vi "StartCCLM.vi"(0 "VISA resource name":refnum<visa-resource-name>, 5 "Device Control-In 2":T1={"Stimulation Parameters"={"Amplitude (mA)"={"A1"=1, "A2"=0, "A3"=0, "A4"=0, "A5"=0, "A6"=0, "A7"=0, "A8"=0}, "Pulse Width (µs)"={"PW1"=20, "PW2"=20, "PW3"=20, "PW4"=20, "PW5"=20, "PW6"=20, "PW7"=20, "PW8"=20}, "Stimulation Mode"={"M1"=0, "M2"=0, "M3"=0, "M4"=0, "M5"=0, "M6"=0, "M7"=0, "M8"=0}}, "Waveform Parameters"={"Low Frequency Factor"=0, "Main Stim Interval [ms]"=8.0, "Interpulse Interval [ms]"=0, "Channel Execution"=0}, "Active channels"={"C1"=FALSE, "C2"=FALSE, "C3"=FALSE, "C4"=FALSE, "C5"=FALSE, "C6"=FALSE, "C7"=FALSE, "C8"=FALSE}, "LF Active Channels"={"LF1"=FALSE, "LF2"=FALSE, "LF3"=FALSE, "LF4"=FALSE, "LF5"=FALSE, "LF6"=FALSE, "LF7"=FALSE, "LF8"=FALSE}, "Device Control"={"VISA resource name"=""}} {"Stimulation Parameters"."Amplitude (mA)"."A1" max=130; "Stimulation Parameters"."Amplitude (mA)"."A2" max=130; "Stimulation Parameters"."Amplitude (mA)"."A3" max=130; "Stimulation Parameters"."Amplitude (mA)"."A4" max=130; "Stimulation Parameters"."Amplitude (mA)"."A5" max=130; "Stimulation Parameters"."Amplitude (mA)"."A6" max=130; "Stimulation Parameters"."Amplitude (mA)"."A7" max=130; "Stimulation Parameters"."Amplitude (mA)"."A8" max=130; "Stimulation Parameters"."Pulse Width (µs)"."PW1" min=20 max=500; "Stimulation Parameters"."Pulse Width (µs)"."PW2" min=20 max=500; "Stimulation Parameters"."Pulse Width (µs)"."PW3" min=20 max=500; "Stimulation Parameters"."Pulse Width (µs)"."PW4" min=20 max=500; "Stimulation Parameters"."Pulse Width (µs)"."PW5" min=20 max=500; "Stimulation Parameters"."Pulse Width (µs)"."PW6" min=20 max=500; "Stimulation Parameters"."Pulse Width (µs)"."PW7" min=20 max=500; "Stimulation Parameters"."Pulse Width (µs)"."PW8" min=20 max=500; "Stimulation Parameters"."Stimulation Mode"."M8" items=["Singlet", "Doublet", "Triplet"]; "Stimulation Parameters"."Stimulation Mode"."M7" items=["Singlet", "Doublet", "Triplet"]; "Stimulation Parameters"."Stimulation Mode"."M6" items=["Singlet", "Doublet", "Triplet"]; "Stimulation Parameters"."Stimulation Mode"."M5" items=["Singlet", "Doublet", "Triplet"]; "Stimulation Parameters"."Stimulation Mode"."M4" items=["Singlet", "Doublet", "Triplet"]; "Stimulation Parameters"."Stimulation Mode"."M3" items=["Singlet", "Doublet", "Triplet"]; "Stimulation Parameters"."Stimulation Mode"."M2" items=["Singlet", "Doublet", "Triplet"]; "Stimulation Parameters"."Stimulation Mode"."M1" items=["Singlet", "Doublet", "Triplet"]; "Waveform Parameters"."Channel Execution" items=["Fixed Interval", "ASAP"]}, 7 "StimInitializationEnable":bool=TRUE, 11 "error in (no error)":errorcluster) -> (4 "VISA resource name out":refnum<visa-resource-name>, 8 "Stimulation Started":bool=TRUE, 15 "error out":errorcluster)   [LabVIEW 2020]
uses:
  Type Defs/rs2_ctrl_panel.ctl
panel:
  in  "Boolean":bool
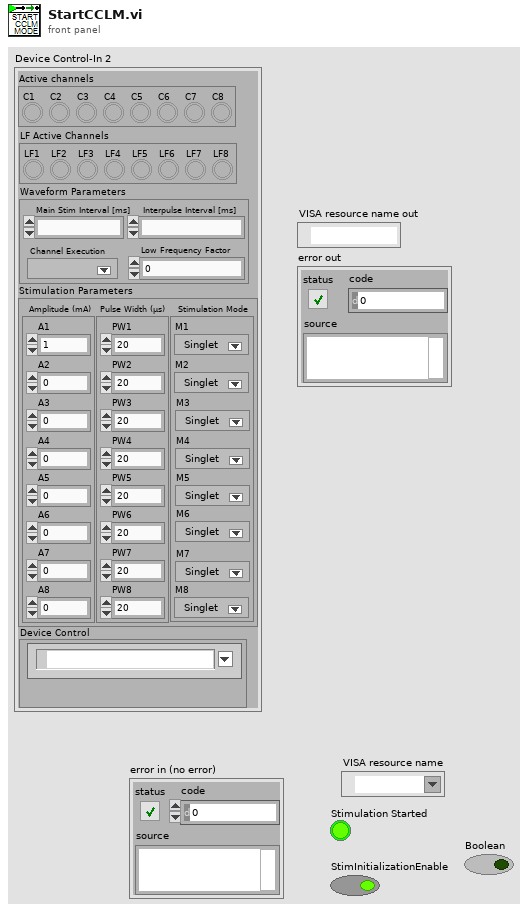
[diagram p1: front panel]
types:
  T1 = typedef "rs2_ctrl_panel.ctl" = cluster{"Stimulation Parameters":cluster{"Amplitude (mA)":cluster{"A1":u8, "A2":u8, "A3":u8, "A4":u8, "A5":u8, "A6":u8, "A7":u8, "A8":u8}, "Pulse Width (µs)":cluster{"PW1":u16, "PW2":u16, "PW3":u16, "PW4":u16, "PW5":u16, "PW6":u16, "PW7":u16, "PW8":u16}, "Stimulation Mode":cluster{"M1":u8, "M2":u8, "M3":u8, "M4":u8, "M5":u8, "M6":u8, "M7":u8, "M8":u8}}, "Waveform Parameters":cluster{"Low Frequency Factor":u8, "Main Stim Interval [ms]":fxp<+,32,11>, "Interpulse Interval [ms]":u8, "Channel Execution":u8}, "Active channels":cluster{"C1":bool, "C2":bool, "C3":bool, "C4":bool, "C5":bool, "C6":bool, "C7":bool, "C8":bool}, "LF Active Channels":cluster{"LF1":bool, "LF2":bool, "LF3":bool, "LF4":bool, "LF5":bool, "LF6":bool, "LF7":bool, "LF8":bool}, "Device Control":cluster{"VISA resource name":refnum<visa-resource-name>}}
  T2 = cluster{"C1":bool, "C2":bool, "C3":bool, "C4":bool, "C5":bool, "C6":bool, "C7":bool, "C8":bool}
  T3 = cluster{"Amplitude (mA)":cluster{"A1":u8, "A2":u8, "A3":u8, "A4":u8, "A5":u8, "A6":u8, "A7":u8, "A8":u8}, "Pulse Width (µs)":cluster{"PW1":u16, "PW2":u16, "PW3":u16, "PW4":u16, "PW5":u16, "PW6":u16, "PW7":u16, "PW8":u16}, "Stimulation Mode":cluster{"M1":u8, "M2":u8, "M3":u8, "M4":u8, "M5":u8, "M6":u8, "M7":u8, "M8":u8}}
  T4 = cluster{"A1":u8, "A2":u8, "A3":u8, "A4":u8, "A5":u8, "A6":u8, "A7":u8, "A8":u8}
  T5 = cluster{"PW1":u16, "PW2":u16, "PW3":u16, "PW4":u16, "PW5":u16, "PW6":u16, "PW7":u16, "PW8":u16}
  T6 = cluster{"M1":u8, "M2":u8, "M3":u8, "M4":u8, "M5":u8, "M6":u8, "M7":u8, "M8":u8}
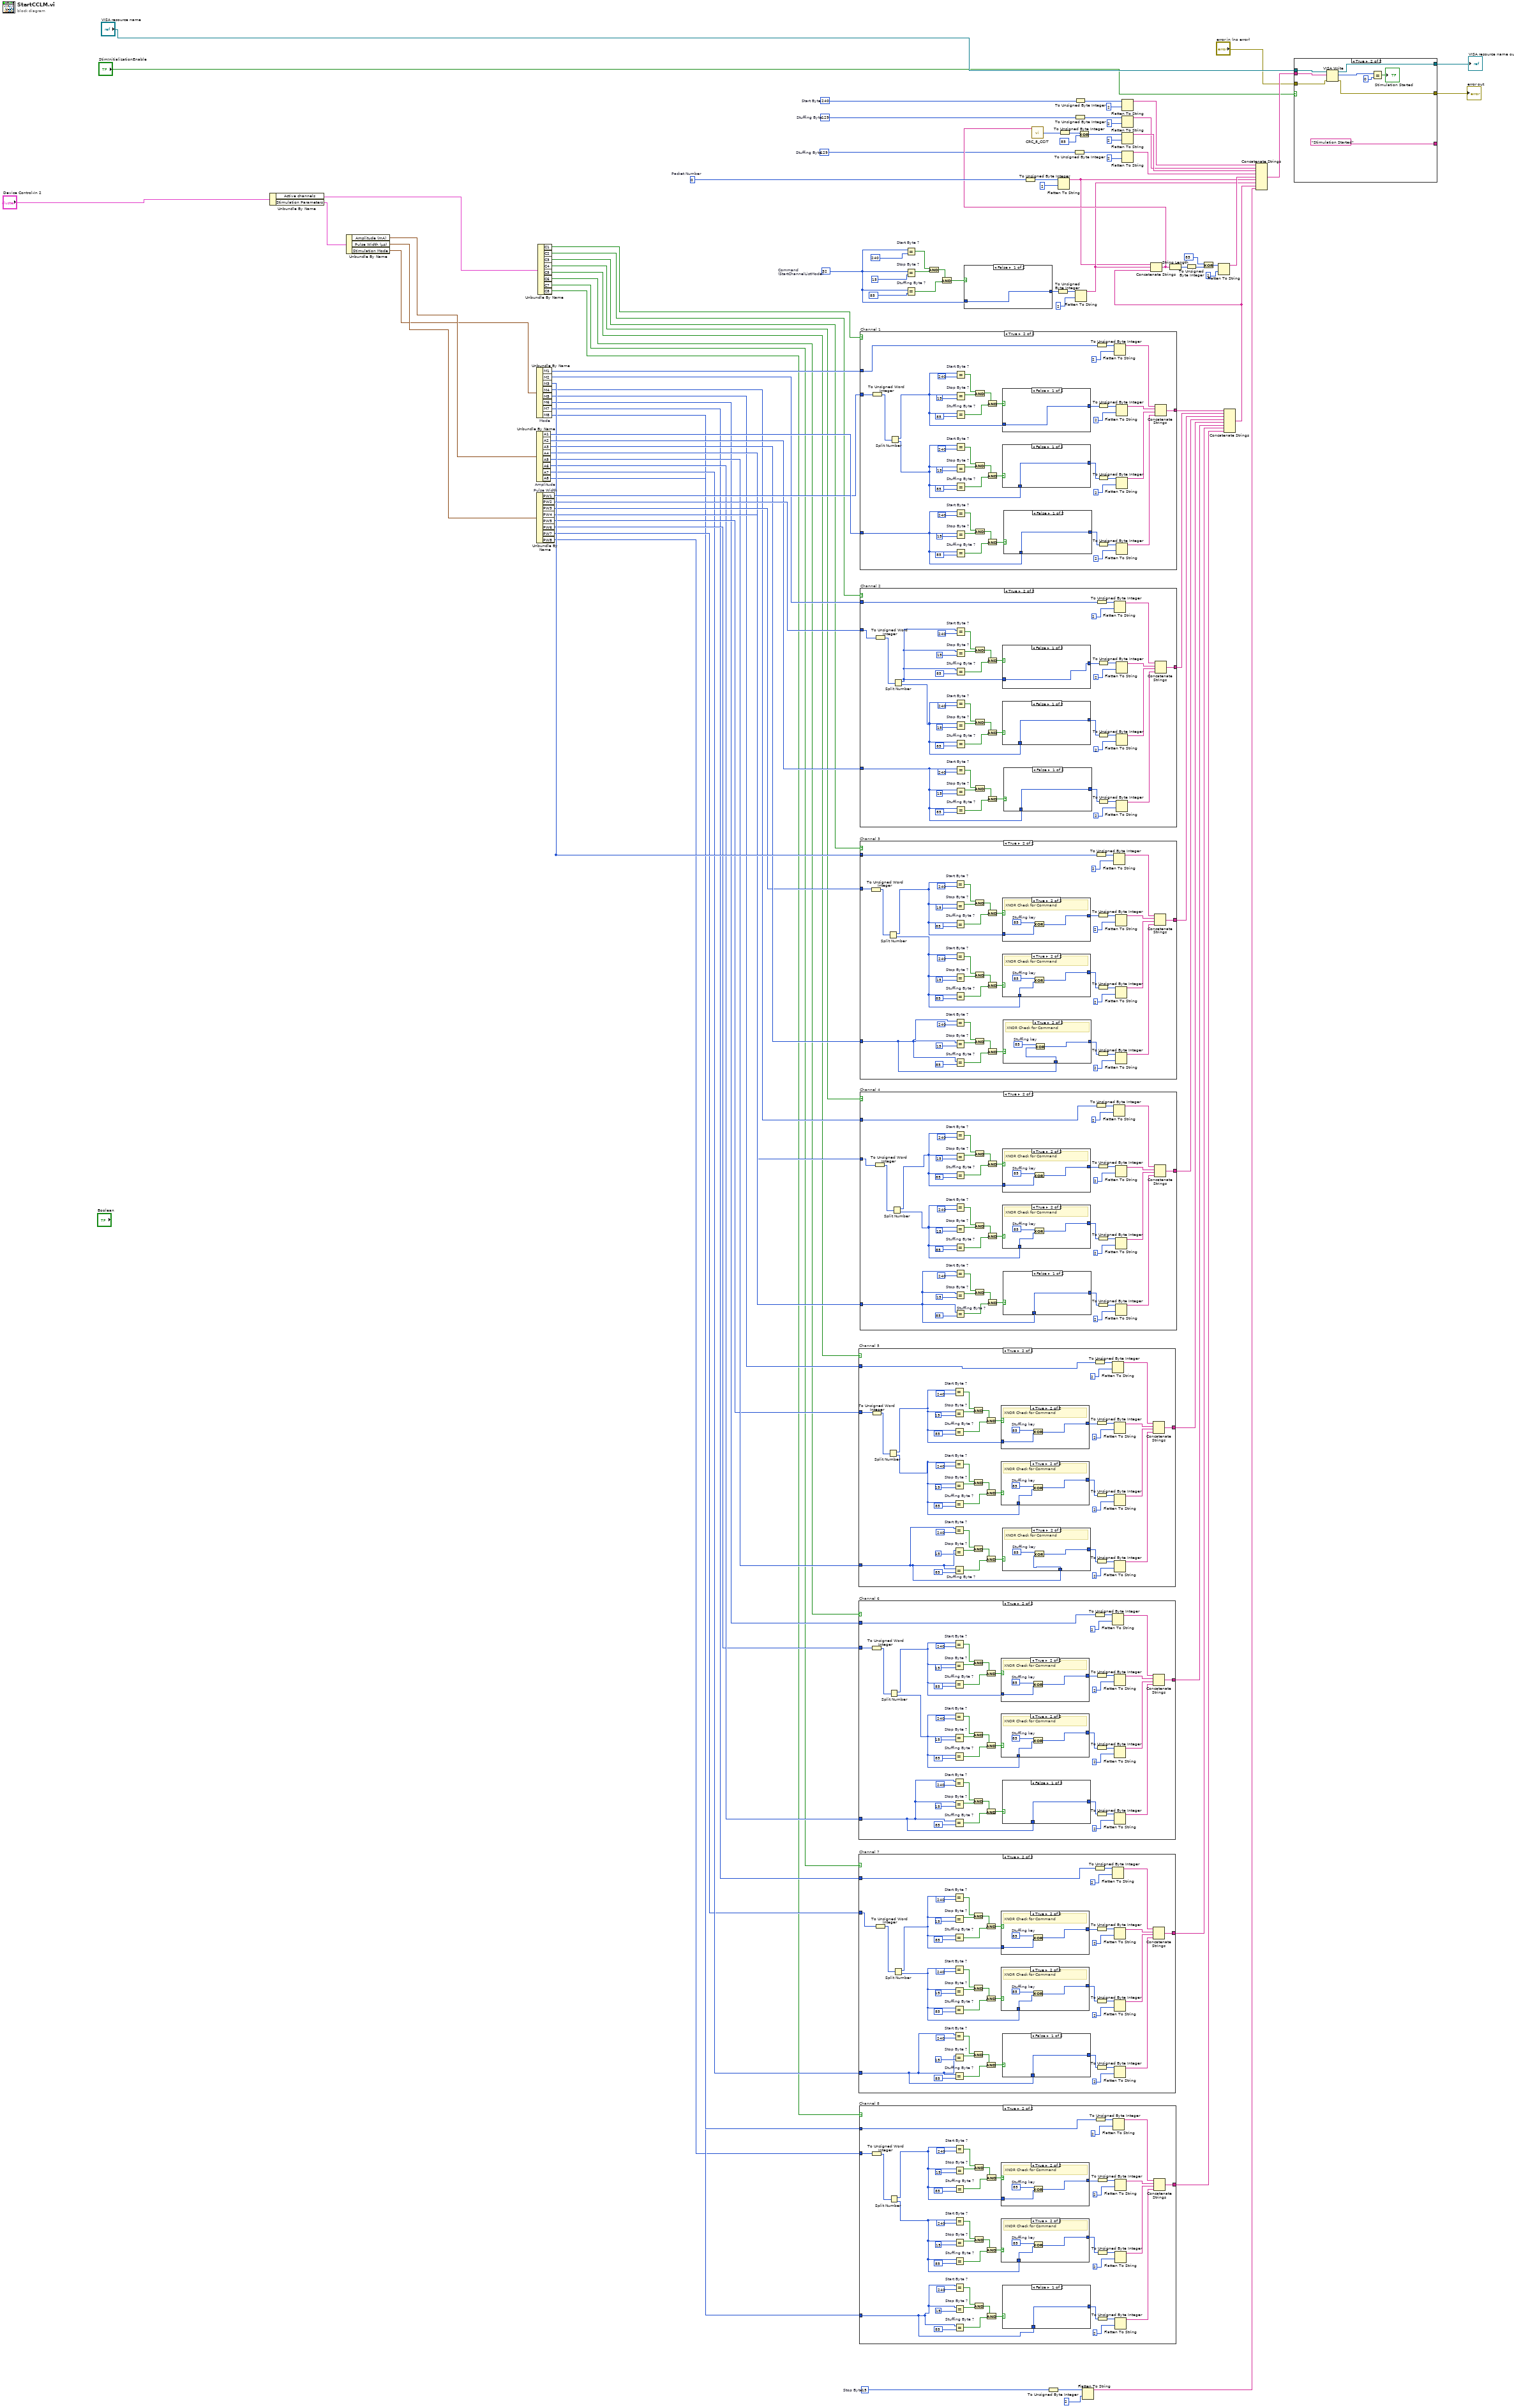
[diagram p0: block diagram]
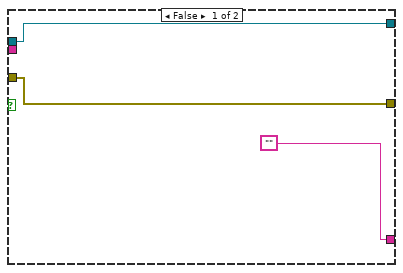
[diagram p2: hidden frame]
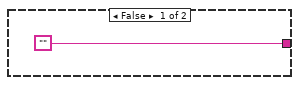
[diagram p3: hidden frame]
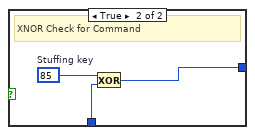
[diagram p4: hidden frame]
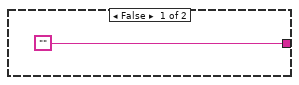
[diagram p7: hidden frame]
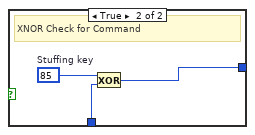
[diagram p8: hidden frame]
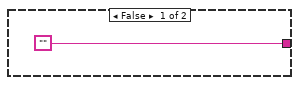
[diagram p11: hidden frame]
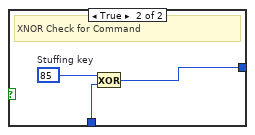
[diagram p12: hidden frame]
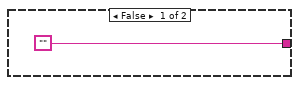
[diagram p15: hidden frame]
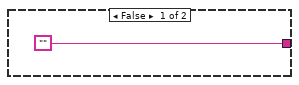
[diagram p19: hidden frame]
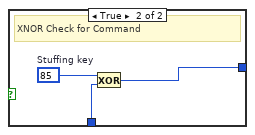
[diagram p20: hidden frame]
diagram:
  w99 = u8 0  # Packet Number
  w63 = 15  # Stop Byte
  w66 = 129  # Stuffing Byte
  w67 = 129  # Stuffing Byte
  w65 = 240  # Start Byte
  w81 = 32  # Command (StartChannelListMode)
  n1 = Unbundle By Name("Device Control-In 2") -> ("Active channels"=w5:T2, "Stimulation Parameters"=w4:T3)
  n2 = Unbundle By Name(w4) -> ("Amplitude (mA)"=w3:T4, "Pulse Width (µs)"=w2:T5, "Stimulation Mode"=w1:T6)
  n3 = Unbundle By Name "Mode"(w1) -> ("M1"=w41:u8, "M2"=w40:u8, "M3"=w37:u8, "M4"=w34:u8, "M5"=w31:u8, "M6"=w28:u8, "M7"=w25:u8, "M8"=w22:u8)
  n4 = Unbundle By Name "Amplitude"(w3) -> ("A1"=w43:u8, "A2"=w38:u8, "A3"=w36:u8, "A4"=w33:u8, "A5"=w30:u8, "A6"=w27:u8, "A7"=w24:u8, "A8"=w21:u8)
  n5 = Unbundle By Name "Pulse Width"(w2) -> ("PW1"=w42:u16, "PW2"=w39:u16, "PW3"=w35:u16, "PW4"=w32:u16, "PW5"=w29:u16, "PW6"=w26:u16, "PW7"=w23:u16, "PW8"=w20:u16)
  n6 = Unbundle By Name(w5) -> ("C1"=w19:bool, "C2"=w18:bool, "C3"=w17:bool, "C4"=w16:bool, "C5"=w15:bool, "C6"=w14:bool, "C7"=w13:bool, "C8"=w12:bool)
  n7 = case "Channel 5" shown="True" w15 {
    tunnel: ["" w107] -> w47
    tunnel: w31 -> [_ w106]
    tunnel: w30 -> [_ w101]
    tunnel: w29 -> [_ w104]
    frame False {
    }
    frame True {
      n8 = To Unsigned Word Integer(number=w104) -> (unsigned 16bit integer=w105:u16)
      n9 = Split Number(x=w105) -> (hi(x)=w103:u8, lo(x)=w102:u8)
      n10 = Equal? "Start Byte ?"(x=w103, y=240 ("IntAck")) -> (x = y?=w136:bool)
      n11 = Equal? "Stop Byte ?"(x=w103, y=15 ("IntAck")) -> (x = y?=w137:bool)
      n12 = Equal? "Stuffing Byte ?"(x=w103, y=85 ("IntAck")) -> (x = y?=w139:bool)
      n13 = Equal? "Start Byte ?"(x=w102, y=240 ("IntAck")) -> (x = y?=w125:bool)
      n14 = Equal? "Stop Byte ?"(x=w102, y=15 ("IntAck")) -> (x = y?=w126:bool)
      n15 = Equal? "Stuffing Byte ?"(x=w102, y=85 ("IntAck")) -> (x = y?=w128:bool)
      n16 = Equal? "Start Byte ?"(x=w101, y=240 ("IntAck")) -> (x = y?=w114:bool)
      n17 = Equal? "Stop Byte ?"(x=w101, y=15 ("IntAck")) -> (x = y?=w115:bool)
      n18 = Equal? "Stuffing Byte ?"(x=w101, y=85 ("IntAck")) -> (x = y?=w117:bool)
      n19 = And(x=w136, y=w137) -> (x .and. y?=w138:bool)
      n20 = And(x=w125, y=w126) -> (x .and. y?=w127:bool)
      n21 = And(x=w114, y=w115) -> (x .and. y?=w116:bool)
      n22 = And(x=w138, y=w139) -> (x .and. y?=w140:bool)
      n23 = And(x=w127, y=w128) -> (x .and. y?=w129:bool)
      n24 = And(x=w116, y=w117) -> (x .and. y?=w118:bool)
      n25 = case shown="True" w140 {
        tunnel: w103 -> [w155 w156]
        tunnel: [w155 w157] -> w145
        frame False {
        }
        frame True {
          w158 = 85  # Stuffing key
          # "XNOR Check for Command"
          n26 = Exclusive Or(1:w156, 2:w158) -> (0:w157:i32)
        }
      }
      n27 = case shown="True" w129 {
        tunnel: w102 -> [w151 w152]
        tunnel: [w151 w153] -> w134
        frame False {
        }
        frame True {
          w154 = 85  # Stuffing key
          # "XNOR Check for Command"
          n28 = Exclusive Or(1:w152, 2:w154) -> (0:w153:i32)
        }
      }
      n29 = case shown="True" w118 {
        tunnel: [w147 w149] -> w123
        tunnel: w101 -> [w147 w148]
        frame False {
        }
        frame True {
          w150 = 85  # Stuffing key
          # "XNOR Check for Command"
          n30 = Exclusive Or(1:w148, 2:w150) -> (0:w149:i32)
        }
      }
      n31 = To Unsigned Byte Integer(number=w106) -> (unsigned 8bit integer=w113:u8)
      n32 = To Unsigned Byte Integer(number=w145) -> (unsigned 8bit integer=w146:u8)
      n33 = To Unsigned Byte Integer(number=w134) -> (unsigned 8bit integer=w135:u8)
      n34 = To Unsigned Byte Integer(number=w123) -> (unsigned 8bit integer=w124:u8)
      n35 = Flatten To String(anything=w113, byte order (0:big-endian, network order)=2) -> (data string=w111:string)  [unwired: 2 in, 2 out]
      n36 = Flatten To String(anything=w146, byte order (0:big-endian, network order)=2) -> (data string=w110:string)  [unwired: 2 in, 2 out]
      n37 = Flatten To String(anything=w135, byte order (0:big-endian, network order)=2) -> (data string=w109:string)  [unwired: 2 in, 2 out]
      n38 = Flatten To String(anything=w124, byte order (0:big-endian, network order)=2) -> (data string=w108:string)  [unwired: 2 in, 2 out]
      n39 = Concatenate Strings(w111, w110, w109, w108) -> (w107:string)
    }
  }
  n40 = case "Channel 6" shown="True" w14 {
    tunnel: ["" w166] -> w46
    tunnel: w26 -> [_ w163]
    tunnel: w27 -> [_ w160]
    tunnel: w28 -> [_ w165]
    frame False {
    }
    frame True {
      n41 = To Unsigned Word Integer(number=w163) -> (unsigned 16bit integer=w164:u16)
      n42 = Split Number(x=w164) -> (hi(x)=w162:u8, lo(x)=w161:u8)
      n43 = Equal? "Start Byte ?"(x=w162, y=240 ("IntAck")) -> (x = y?=w195:bool)
      n44 = Equal? "Stop Byte ?"(x=w162, y=15 ("IntAck")) -> (x = y?=w196:bool)
      n45 = Equal? "Stuffing Byte ?"(x=w162, y=85 ("IntAck")) -> (x = y?=w198:bool)
      n46 = Equal? "Start Byte ?"(x=w161, y=240 ("IntAck")) -> (x = y?=w184:bool)
      n47 = Equal? "Stop Byte ?"(x=w161, y=15 ("IntAck")) -> (x = y?=w185:bool)
      n48 = Equal? "Stuffing Byte ?"(x=w161, y=85 ("IntAck")) -> (x = y?=w187:bool)
      n49 = Equal? "Start Byte ?"(x=w160, y=240 ("IntAck")) -> (x = y?=w173:bool)
      n50 = Equal? "Stop Byte ?"(x=w160, y=15 ("IntAck")) -> (x = y?=w174:bool)
      n51 = Equal? "Stuffing Byte ?"(x=w160, y=85 ("IntAck")) -> (x = y?=w176:bool)
      n52 = And(x=w195, y=w196) -> (x .and. y?=w197:bool)
      n53 = And(x=w184, y=w185) -> (x .and. y?=w186:bool)
      n54 = And(x=w173, y=w174) -> (x .and. y?=w175:bool)
      n55 = And(x=w197, y=w198) -> (x .and. y?=w199:bool)
      n56 = And(x=w186, y=w187) -> (x .and. y?=w188:bool)
      n57 = And(x=w175, y=w176) -> (x .and. y?=w177:bool)
      n58 = case shown="True" w199 {
        tunnel: w162 -> [w214 w215]
        tunnel: [w214 w216] -> w204
        frame False {
        }
        frame True {
          w217 = 85  # Stuffing key
          # "XNOR Check for Command"
          n59 = Exclusive Or(1:w215, 2:w217) -> (0:w216:i32)
        }
      }
      n60 = case shown="True" w188 {
        tunnel: w161 -> [w210 w211]
        tunnel: [w210 w212] -> w193
        frame False {
        }
        frame True {
          w213 = 85  # Stuffing key
          # "XNOR Check for Command"
          n61 = Exclusive Or(1:w211, 2:w213) -> (0:w212:i32)
        }
      }
      n62 = case shown="False" w177 {
        tunnel: [w206 w208] -> w182
        tunnel: w160 -> [w206 w207]
        frame False {
        }
        frame True {
          w209 = 85  # Stuffing key
          # "XNOR Check for Command"
          n63 = Exclusive Or(1:w207, 2:w209) -> (0:w208:i32)
        }
      }
      n64 = To Unsigned Byte Integer(number=w165) -> (unsigned 8bit integer=w172:u8)
      n65 = To Unsigned Byte Integer(number=w204) -> (unsigned 8bit integer=w205:u8)
      n66 = To Unsigned Byte Integer(number=w193) -> (unsigned 8bit integer=w194:u8)
      n67 = To Unsigned Byte Integer(number=w182) -> (unsigned 8bit integer=w183:u8)
      n68 = Flatten To String(anything=w172, byte order (0:big-endian, network order)=2) -> (data string=w170:string)  [unwired: 2 in, 2 out]
      n69 = Flatten To String(anything=w205, byte order (0:big-endian, network order)=2) -> (data string=w169:string)  [unwired: 2 in, 2 out]
      n70 = Flatten To String(anything=w194, byte order (0:big-endian, network order)=2) -> (data string=w168:string)  [unwired: 2 in, 2 out]
      n71 = Flatten To String(anything=w183, byte order (0:big-endian, network order)=2) -> (data string=w167:string)  [unwired: 2 in, 2 out]
      n72 = Concatenate Strings(w170, w169, w168, w167) -> (w166:string)
    }
  }
  n73 = case "Channel 7" shown="True" w13 {
    tunnel: ["" w225] -> w45
    tunnel: w23 -> [_ w222]
    tunnel: w24 -> [_ w219]
    tunnel: w25 -> [_ w224]
    frame False {
    }
    frame True {
      n74 = To Unsigned Word Integer(number=w222) -> (unsigned 16bit integer=w223:u16)
      n75 = Split Number(x=w223) -> (hi(x)=w221:u8, lo(x)=w220:u8)
      n76 = Equal? "Start Byte ?"(x=w221, y=240 ("IntAck")) -> (x = y?=w254:bool)
      n77 = Equal? "Stop Byte ?"(x=w221, y=15 ("IntAck")) -> (x = y?=w255:bool)
      n78 = Equal? "Stuffing Byte ?"(x=w221, y=85 ("IntAck")) -> (x = y?=w257:bool)
      n79 = Equal? "Start Byte ?"(x=w220, y=240 ("IntAck")) -> (x = y?=w243:bool)
      n80 = Equal? "Stop Byte ?"(x=w220, y=15 ("IntAck")) -> (x = y?=w244:bool)
      n81 = Equal? "Stuffing Byte ?"(x=w220, y=85 ("IntAck")) -> (x = y?=w246:bool)
      n82 = Equal? "Start Byte ?"(x=w219, y=240 ("IntAck")) -> (x = y?=w232:bool)
      n83 = Equal? "Stop Byte ?"(x=w219, y=15 ("IntAck")) -> (x = y?=w233:bool)
      n84 = Equal? "Stuffing Byte ?"(x=w219, y=85 ("IntAck")) -> (x = y?=w235:bool)
      n85 = And(x=w254, y=w255) -> (x .and. y?=w256:bool)
      n86 = And(x=w243, y=w244) -> (x .and. y?=w245:bool)
      n87 = And(x=w232, y=w233) -> (x .and. y?=w234:bool)
      n88 = And(x=w256, y=w257) -> (x .and. y?=w258:bool)
      n89 = And(x=w245, y=w246) -> (x .and. y?=w247:bool)
      n90 = And(x=w234, y=w235) -> (x .and. y?=w236:bool)
      n91 = case shown="True" w258 {
        tunnel: w221 -> [w273 w274]
        tunnel: [w273 w275] -> w263
        frame False {
        }
        frame True {
          w276 = 85  # Stuffing key
          # "XNOR Check for Command"
          n92 = Exclusive Or(1:w274, 2:w276) -> (0:w275:i32)
        }
      }
      n93 = case shown="True" w247 {
        tunnel: w220 -> [w269 w270]
        tunnel: [w269 w271] -> w252
        frame False {
        }
        frame True {
          w272 = 85  # Stuffing key
          # "XNOR Check for Command"
          n94 = Exclusive Or(1:w270, 2:w272) -> (0:w271:i32)
        }
      }
      n95 = case shown="False" w236 {
        tunnel: [w265 w267] -> w241
        tunnel: w219 -> [w265 w266]
        frame False {
        }
        frame True {
          w268 = 85  # Stuffing key
          # "XNOR Check for Command"
          n96 = Exclusive Or(1:w266, 2:w268) -> (0:w267:i32)
        }
      }
      n97 = To Unsigned Byte Integer(number=w224) -> (unsigned 8bit integer=w231:u8)
      n98 = To Unsigned Byte Integer(number=w263) -> (unsigned 8bit integer=w264:u8)
      n99 = To Unsigned Byte Integer(number=w252) -> (unsigned 8bit integer=w253:u8)
      n100 = To Unsigned Byte Integer(number=w241) -> (unsigned 8bit integer=w242:u8)
      n101 = Flatten To String(anything=w231, byte order (0:big-endian, network order)=2) -> (data string=w229:string)  [unwired: 2 in, 2 out]
      n102 = Flatten To String(anything=w264, byte order (0:big-endian, network order)=2) -> (data string=w228:string)  [unwired: 2 in, 2 out]
      n103 = Flatten To String(anything=w253, byte order (0:big-endian, network order)=2) -> (data string=w227:string)  [unwired: 2 in, 2 out]
      n104 = Flatten To String(anything=w242, byte order (0:big-endian, network order)=2) -> (data string=w226:string)  [unwired: 2 in, 2 out]
      n105 = Concatenate Strings(w229, w228, w227, w226) -> (w225:string)
    }
  }
  n106 = case "Channel 8" shown="True" w12 {
    tunnel: ["" w284] -> w44
    tunnel: w20 -> [_ w281]
    tunnel: w21 -> [_ w278]
    tunnel: w22 -> [_ w283]
    frame False {
    }
    frame True {
      n107 = To Unsigned Word Integer(number=w281) -> (unsigned 16bit integer=w282:u16)
      n108 = Split Number(x=w282) -> (hi(x)=w280:u8, lo(x)=w279:u8)
      n109 = Equal? "Start Byte ?"(x=w280, y=240 ("IntAck")) -> (x = y?=w313:bool)
      n110 = Equal? "Stop Byte ?"(x=w280, y=15 ("IntAck")) -> (x = y?=w314:bool)
      n111 = Equal? "Stuffing Byte ?"(x=w280, y=85 ("IntAck")) -> (x = y?=w316:bool)
      n112 = Equal? "Start Byte ?"(x=w279, y=240 ("IntAck")) -> (x = y?=w302:bool)
      n113 = Equal? "Stop Byte ?"(x=w279, y=15 ("IntAck")) -> (x = y?=w303:bool)
      n114 = Equal? "Stuffing Byte ?"(x=w279, y=85 ("IntAck")) -> (x = y?=w305:bool)
      n115 = Equal? "Start Byte ?"(x=w278, y=240 ("IntAck")) -> (x = y?=w291:bool)
      n116 = Equal? "Stop Byte ?"(x=w278, y=15 ("IntAck")) -> (x = y?=w292:bool)
      n117 = Equal? "Stuffing Byte ?"(x=w278, y=85 ("IntAck")) -> (x = y?=w294:bool)
      n118 = And(x=w313, y=w314) -> (x .and. y?=w315:bool)
      n119 = And(x=w302, y=w303) -> (x .and. y?=w304:bool)
      n120 = And(x=w291, y=w292) -> (x .and. y?=w293:bool)
      n121 = And(x=w315, y=w316) -> (x .and. y?=w317:bool)
      n122 = And(x=w304, y=w305) -> (x .and. y?=w306:bool)
      n123 = And(x=w293, y=w294) -> (x .and. y?=w295:bool)
      n124 = case shown="True" w317 {
        tunnel: w280 -> [w332 w333]
        tunnel: [w332 w334] -> w322
        frame False {
        }
        frame True {
          w335 = 85  # Stuffing key
          # "XNOR Check for Command"
          n125 = Exclusive Or(1:w333, 2:w335) -> (0:w334:i32)
        }
      }
      n126 = case shown="True" w306 {
        tunnel: w279 -> [w328 w329]
        tunnel: [w328 w330] -> w311
        frame False {
        }
        frame True {
          w331 = 85  # Stuffing key
          # "XNOR Check for Command"
          n127 = Exclusive Or(1:w329, 2:w331) -> (0:w330:i32)
        }
      }
      n128 = case shown="False" w295 {
        tunnel: [w324 w326] -> w300
        tunnel: w278 -> [w324 w325]
        frame False {
        }
        frame True {
          w327 = 85  # Stuffing key
          # "XNOR Check for Command"
          n129 = Exclusive Or(1:w325, 2:w327) -> (0:w326:i32)
        }
      }
      n130 = To Unsigned Byte Integer(number=w283) -> (unsigned 8bit integer=w290:u8)
      n131 = To Unsigned Byte Integer(number=w322) -> (unsigned 8bit integer=w323:u8)
      n132 = To Unsigned Byte Integer(number=w311) -> (unsigned 8bit integer=w312:u8)
      n133 = To Unsigned Byte Integer(number=w300) -> (unsigned 8bit integer=w301:u8)
      n134 = Flatten To String(anything=w290, byte order (0:big-endian, network order)=2) -> (data string=w288:string)  [unwired: 2 in, 2 out]
      n135 = Flatten To String(anything=w323, byte order (0:big-endian, network order)=2) -> (data string=w287:string)  [unwired: 2 in, 2 out]
      n136 = Flatten To String(anything=w312, byte order (0:big-endian, network order)=2) -> (data string=w286:string)  [unwired: 2 in, 2 out]
      n137 = Flatten To String(anything=w301, byte order (0:big-endian, network order)=2) -> (data string=w285:string)  [unwired: 2 in, 2 out]
      n138 = Concatenate Strings(w288, w287, w286, w285) -> (w284:string)
    }
  }
  n139 = case "Channel 3" shown="True" w17 {
    tunnel: ["" w343] -> w49
    tunnel: w37 -> [_ _]
    tunnel: w37 -> [_ w342]
    tunnel: w36 -> [_ w337]
    tunnel: w35 -> [_ w340]
    frame False {
    }
    frame True {
      n140 = To Unsigned Word Integer(number=w340) -> (unsigned 16bit integer=w341:u16)
      n141 = Split Number(x=w341) -> (hi(x)=w339:u8, lo(x)=w338:u8)
      n142 = Equal? "Start Byte ?"(x=w339, y=240 ("IntAck")) -> (x = y?=w372:bool)
      n143 = Equal? "Stop Byte ?"(x=w339, y=15 ("IntAck")) -> (x = y?=w373:bool)
      n144 = Equal? "Stuffing Byte ?"(x=w339, y=85 ("IntAck")) -> (x = y?=w375:bool)
      n145 = Equal? "Start Byte ?"(x=w338, y=240 ("IntAck")) -> (x = y?=w361:bool)
      n146 = Equal? "Stop Byte ?"(x=w338, y=15 ("IntAck")) -> (x = y?=w362:bool)
      n147 = Equal? "Stuffing Byte ?"(x=w338, y=85 ("IntAck")) -> (x = y?=w364:bool)
      n148 = Equal? "Start Byte ?"(x=w337, y=240 ("IntAck")) -> (x = y?=w350:bool)
      n149 = Equal? "Stop Byte ?"(x=w337, y=15 ("IntAck")) -> (x = y?=w351:bool)
      n150 = Equal? "Stuffing Byte ?"(x=w337, y=85 ("IntAck")) -> (x = y?=w353:bool)
      n151 = And(x=w372, y=w373) -> (x .and. y?=w374:bool)
      n152 = And(x=w361, y=w362) -> (x .and. y?=w363:bool)
      n153 = And(x=w350, y=w351) -> (x .and. y?=w352:bool)
      n154 = And(x=w374, y=w375) -> (x .and. y?=w376:bool)
      n155 = And(x=w363, y=w364) -> (x .and. y?=w365:bool)
      n156 = And(x=w352, y=w353) -> (x .and. y?=w354:bool)
      n157 = case shown="True" w376 {
        tunnel: w339 -> [w391 w392]
        tunnel: [w391 w393] -> w381
        frame False {
        }
        frame True {
          w394 = 85  # Stuffing key
          # "XNOR Check for Command"
          n158 = Exclusive Or(1:w392, 2:w394) -> (0:w393:i32)
        }
      }
      n159 = case shown="True" w365 {
        tunnel: w338 -> [w387 w388]
        tunnel: [w387 w389] -> w370
        frame False {
        }
        frame True {
          w390 = 85  # Stuffing key
          # "XNOR Check for Command"
          n160 = Exclusive Or(1:w388, 2:w390) -> (0:w389:i32)
        }
      }
      n161 = case shown="True" w354 {
        tunnel: [w383 w385] -> w359
        tunnel: w337 -> [w383 w384]
        frame False {
        }
        frame True {
          w386 = 85  # Stuffing key
          # "XNOR Check for Command"
          n162 = Exclusive Or(1:w384, 2:w386) -> (0:w385:i32)
        }
      }
      n163 = To Unsigned Byte Integer(number=w342) -> (unsigned 8bit integer=w349:u8)
      n164 = To Unsigned Byte Integer(number=w381) -> (unsigned 8bit integer=w382:u8)
      n165 = To Unsigned Byte Integer(number=w370) -> (unsigned 8bit integer=w371:u8)
      n166 = To Unsigned Byte Integer(number=w359) -> (unsigned 8bit integer=w360:u8)
      n167 = Flatten To String(anything=w349, byte order (0:big-endian, network order)=2) -> (data string=w347:string)  [unwired: 2 in, 2 out]
      n168 = Flatten To String(anything=w382, byte order (0:big-endian, network order)=2) -> (data string=w346:string)  [unwired: 2 in, 2 out]
      n169 = Flatten To String(anything=w371, byte order (0:big-endian, network order)=2) -> (data string=w345:string)  [unwired: 2 in, 2 out]
      n170 = Flatten To String(anything=w360, byte order (0:big-endian, network order)=2) -> (data string=w344:string)  [unwired: 2 in, 2 out]
      n171 = Concatenate Strings(w347, w346, w345, w344) -> (w343:string)
    }
  }
  n172 = case "Channel 4" shown="True" w16 {
    tunnel: ["" w402] -> w48
    tunnel: w34 -> [_ w401]
    tunnel: w33 -> [_ w396]
    tunnel: w32 -> [_ w399]
    frame False {
    }
    frame True {
      n173 = To Unsigned Word Integer(number=w399) -> (unsigned 16bit integer=w400:u16)
      n174 = Split Number(x=w400) -> (hi(x)=w398:u8, lo(x)=w397:u8)
      n175 = Equal? "Start Byte ?"(x=w398, y=240 ("IntAck")) -> (x = y?=w431:bool)
      n176 = Equal? "Stop Byte ?"(x=w398, y=15 ("IntAck")) -> (x = y?=w432:bool)
      n177 = Equal? "Stuffing Byte ?"(x=w398, y=85 ("IntAck")) -> (x = y?=w434:bool)
      n178 = Equal? "Start Byte ?"(x=w397, y=240 ("IntAck")) -> (x = y?=w420:bool)
      n179 = Equal? "Stop Byte ?"(x=w397, y=15 ("IntAck")) -> (x = y?=w421:bool)
      n180 = Equal? "Stuffing Byte ?"(x=w397, y=85 ("IntAck")) -> (x = y?=w423:bool)
      n181 = Equal? "Start Byte ?"(x=w396, y=240 ("IntAck")) -> (x = y?=w409:bool)
      n182 = Equal? "Stop Byte ?"(x=w396, y=15 ("IntAck")) -> (x = y?=w410:bool)
      n183 = Equal? "Stuffing Byte ?"(x=w396, y=85 ("IntAck")) -> (x = y?=w412:bool)
      n184 = And(x=w431, y=w432) -> (x .and. y?=w433:bool)
      n185 = And(x=w420, y=w421) -> (x .and. y?=w422:bool)
      n186 = And(x=w409, y=w410) -> (x .and. y?=w411:bool)
      n187 = And(x=w433, y=w434) -> (x .and. y?=w435:bool)
      n188 = And(x=w422, y=w423) -> (x .and. y?=w424:bool)
      n189 = And(x=w411, y=w412) -> (x .and. y?=w413:bool)
      n190 = case shown="True" w435 {
        tunnel: w398 -> [w450 w451]
        tunnel: [w450 w452] -> w440
        frame False {
        }
        frame True {
          w453 = 85  # Stuffing key
          # "XNOR Check for Command"
          n191 = Exclusive Or(1:w451, 2:w453) -> (0:w452:i32)
        }
      }
      n192 = case shown="True" w424 {
        tunnel: w397 -> [w446 w447]
        tunnel: [w446 w448] -> w429
        frame False {
        }
        frame True {
          w449 = 85  # Stuffing key
          # "XNOR Check for Command"
          n193 = Exclusive Or(1:w447, 2:w449) -> (0:w448:i32)
        }
      }
      n194 = case shown="False" w413 {
        tunnel: [w442 w444] -> w418
        tunnel: w396 -> [w442 w443]
        frame False {
        }
        frame True {
          w445 = 85  # Stuffing key
          # "XNOR Check for Command"
          n195 = Exclusive Or(1:w443, 2:w445) -> (0:w444:i32)
        }
      }
      n196 = To Unsigned Byte Integer(number=w401) -> (unsigned 8bit integer=w408:u8)
      n197 = To Unsigned Byte Integer(number=w440) -> (unsigned 8bit integer=w441:u8)
      n198 = To Unsigned Byte Integer(number=w429) -> (unsigned 8bit integer=w430:u8)
      n199 = To Unsigned Byte Integer(number=w418) -> (unsigned 8bit integer=w419:u8)
      n200 = Flatten To String(anything=w408, byte order (0:big-endian, network order)=2) -> (data string=w406:string)  [unwired: 2 in, 2 out]
      n201 = Flatten To String(anything=w441, byte order (0:big-endian, network order)=2) -> (data string=w405:string)  [unwired: 2 in, 2 out]
      n202 = Flatten To String(anything=w430, byte order (0:big-endian, network order)=2) -> (data string=w404:string)  [unwired: 2 in, 2 out]
      n203 = Flatten To String(anything=w419, byte order (0:big-endian, network order)=2) -> (data string=w403:string)  [unwired: 2 in, 2 out]
      n204 = Concatenate Strings(w406, w405, w404, w403) -> (w402:string)
    }
  }
  n205 = case "Channel 1" shown="True" w19 {
    tunnel: ["" w461] -> w51
    tunnel: w43 -> [_ w460]
    tunnel: w42 -> [_ w456]
    tunnel: w41 -> [_ w459]
    frame False {
    }
    frame True {
      n206 = To Unsigned Word Integer(number=w456) -> (unsigned 16bit integer=w455:u16)
      n207 = Split Number(x=w455) -> (hi(x)=w457:u8, lo(x)=w458:u8)
      n208 = Equal? "Start Byte ?"(x=w457, y=240 ("IntAck")) -> (x = y?=w490:bool)
      n209 = Equal? "Stop Byte ?"(x=w457, y=15 ("IntAck")) -> (x = y?=w491:bool)
      n210 = Equal? "Stuffing Byte ?"(x=w457, y=85 ("IntAck")) -> (x = y?=w493:bool)
      n211 = Equal? "Start Byte ?"(x=w458, y=240 ("IntAck")) -> (x = y?=w479:bool)
      n212 = Equal? "Stop Byte ?"(x=w458, y=15 ("IntAck")) -> (x = y?=w480:bool)
      n213 = Equal? "Stuffing Byte ?"(x=w458, y=85 ("IntAck")) -> (x = y?=w482:bool)
      n214 = Equal? "Start Byte ?"(x=w460, y=240 ("IntAck")) -> (x = y?=w468:bool)
      n215 = Equal? "Stop Byte ?"(x=w460, y=15 ("IntAck")) -> (x = y?=w469:bool)
      n216 = Equal? "Stuffing Byte ?"(x=w460, y=85 ("IntAck")) -> (x = y?=w471:bool)
      n217 = And(x=w490, y=w491) -> (x .and. y?=w492:bool)
      n218 = And(x=w479, y=w480) -> (x .and. y?=w481:bool)
      n219 = And(x=w468, y=w469) -> (x .and. y?=w470:bool)
      n220 = And(x=w492, y=w493) -> (x .and. y?=w494:bool)
      n221 = And(x=w481, y=w482) -> (x .and. y?=w483:bool)
      n222 = And(x=w470, y=w471) -> (x .and. y?=w472:bool)
      n223 = case shown="False" w494 {
        tunnel: w457 -> [w509 w510]
        tunnel: [w509 w511] -> w499
        frame False {
        }
        frame True {
          w512 = 85  # Stuffing key
          # "XNOR Check for Command"
          n224 = Exclusive Or(1:w510, 2:w512) -> (0:w511:i32)
        }
      }
      n225 = case shown="False" w483 {
        tunnel: w458 -> [w505 w506]
        tunnel: [w505 w507] -> w488
        frame False {
        }
        frame True {
          w508 = 85  # Stuffing key
          # "XNOR Check for Command"
          n226 = Exclusive Or(1:w506, 2:w508) -> (0:w507:i32)
        }
      }
      n227 = case shown="False" w472 {
        tunnel: w460 -> [w501 w502]
        tunnel: [w501 w503] -> w477
        frame False {
        }
        frame True {
          w504 = 85  # Stuffing key
          # "XNOR Check for Command"
          n228 = Exclusive Or(1:w502, 2:w504) -> (0:w503:i32)
        }
      }
      n229 = To Unsigned Byte Integer(number=w459) -> (unsigned 8bit integer=w467:u8)
      n230 = To Unsigned Byte Integer(number=w499) -> (unsigned 8bit integer=w500:u8)
      n231 = To Unsigned Byte Integer(number=w488) -> (unsigned 8bit integer=w489:u8)
      n232 = To Unsigned Byte Integer(number=w477) -> (unsigned 8bit integer=w478:u8)
      n233 = Flatten To String(anything=w467, byte order (0:big-endian, network order)=2) -> (data string=w465:string)  [unwired: 2 in, 2 out]
      n234 = Flatten To String(anything=w500, byte order (0:big-endian, network order)=2) -> (data string=w464:string)  [unwired: 2 in, 2 out]
      n235 = Flatten To String(anything=w489, byte order (0:big-endian, network order)=2) -> (data string=w463:string)  [unwired: 2 in, 2 out]
      n236 = Flatten To String(anything=w478, byte order (0:big-endian, network order)=2) -> (data string=w462:string)  [unwired: 2 in, 2 out]
      n237 = Concatenate Strings(w465, w464, w463, w462) -> (w461:string)
    }
  }
  n238 = case "Channel 2" shown="True" w18 {
    tunnel: ["" w520] -> w50
    tunnel: w40 -> [_ w519]
    tunnel: w39 -> [_ w516]
    tunnel: w38 -> [_ w518]
    frame False {
    }
    frame True {
      n239 = To Unsigned Word Integer(number=w516) -> (unsigned 16bit integer=w517:u16)
      n240 = Split Number(x=w517) -> (hi(x)=w514:u8, lo(x)=w515:u8)
      n241 = Equal? "Start Byte ?"(x=w514, y=240 ("IntAck")) -> (x = y?=w549:bool)
      n242 = Equal? "Stop Byte ?"(x=w514, y=15 ("IntAck")) -> (x = y?=w550:bool)
      n243 = Equal? "Stuffing Byte ?"(x=w514, y=85 ("IntAck")) -> (x = y?=w552:bool)
      n244 = Equal? "Start Byte ?"(x=w515, y=240 ("IntAck")) -> (x = y?=w538:bool)
      n245 = Equal? "Stop Byte ?"(x=w515, y=15 ("IntAck")) -> (x = y?=w539:bool)
      n246 = Equal? "Stuffing Byte ?"(x=w515, y=85 ("IntAck")) -> (x = y?=w541:bool)
      n247 = Equal? "Start Byte ?"(x=w518, y=240 ("IntAck")) -> (x = y?=w527:bool)
      n248 = Equal? "Stop Byte ?"(x=w518, y=15 ("IntAck")) -> (x = y?=w528:bool)
      n249 = Equal? "Stuffing Byte ?"(x=w518, y=85 ("IntAck")) -> (x = y?=w530:bool)
      n250 = And(x=w549, y=w550) -> (x .and. y?=w551:bool)
      n251 = And(x=w538, y=w539) -> (x .and. y?=w540:bool)
      n252 = And(x=w527, y=w528) -> (x .and. y?=w529:bool)
      n253 = And(x=w551, y=w552) -> (x .and. y?=w553:bool)
      n254 = And(x=w540, y=w541) -> (x .and. y?=w542:bool)
      n255 = And(x=w529, y=w530) -> (x .and. y?=w531:bool)
      n256 = case shown="False" w553 {
        tunnel: [w568 w570] -> w558
        tunnel: w514 -> [w568 w569]
        frame False {
        }
        frame True {
          w571 = 85  # Stuffing key
          # "XNOR Check for Command"
          n257 = Exclusive Or(1:w569, 2:w571) -> (0:w570:i32)
        }
      }
      n258 = case shown="False" w542 {
        tunnel: w515 -> [w564 w565]
        tunnel: [w564 w566] -> w547
        frame False {
        }
        frame True {
          w567 = 85  # Stuffing key
          # "XNOR Check for Command"
          n259 = Exclusive Or(1:w565, 2:w567) -> (0:w566:i32)
        }
      }
      n260 = case shown="False" w531 {
        tunnel: w518 -> [w560 w561]
        tunnel: [w560 w562] -> w536
        frame False {
        }
        frame True {
          w563 = 85  # Stuffing key
          # "XNOR Check for Command"
          n261 = Exclusive Or(1:w561, 2:w563) -> (0:w562:i32)
        }
      }
      n262 = To Unsigned Byte Integer(number=w519) -> (unsigned 8bit integer=w526:u8)
      n263 = To Unsigned Byte Integer(number=w558) -> (unsigned 8bit integer=w559:u8)
      n264 = To Unsigned Byte Integer(number=w547) -> (unsigned 8bit integer=w548:u8)
      n265 = To Unsigned Byte Integer(number=w536) -> (unsigned 8bit integer=w537:u8)
      n266 = Flatten To String(anything=w526, byte order (0:big-endian, network order)=2) -> (data string=w524:string)  [unwired: 2 in, 2 out]
      n267 = Flatten To String(anything=w559, byte order (0:big-endian, network order)=2) -> (data string=w523:string)  [unwired: 2 in, 2 out]
      n268 = Flatten To String(anything=w548, byte order (0:big-endian, network order)=2) -> (data string=w522:string)  [unwired: 2 in, 2 out]
      n269 = Flatten To String(anything=w537, byte order (0:big-endian, network order)=2) -> (data string=w521:string)  [unwired: 2 in, 2 out]
      n270 = Concatenate Strings(w524, w523, w522, w521) -> (w520:string)
    }
  }
  n271 = Equal? "Start Byte ?"(x=w81, y=240 ("IntAck")) -> (x = y?=w54:bool)
  n272 = Equal? "Stop Byte ?"(x=w81, y=15 ("IntAck")) -> (x = y?=w55:bool)
  n273 = Equal? "Stuffing Byte ?"(x=w81, y=85 ("IntAck")) -> (x = y?=w57:bool)
  n274 = And(x=w54, y=w55) -> (x .and. y?=w56:bool)
  n275 = And(x=w56, y=w57) -> (x .and. y?=w58:bool)
  n276 = case shown="False" w58 {
    tunnel: w81 -> [w572 w575]
    tunnel: [w572 w573] -> w82
    frame False {
    }
    frame True {
      w574 = 85  # Stuffing key
      # "XNOR Check for Command"
      n277 = Exclusive Or(1:w575, 2:w574) -> (0:w573:i32)
    }
  }
  n278 = To Unsigned Byte Integer(number=w99) -> (unsigned 8bit integer=w89:u8)
  n279 = To Unsigned Byte Integer(number=w63) -> (unsigned 8bit integer=w64:u8)
  n280 = To Unsigned Byte Integer(number=w82) -> (unsigned 8bit integer=w88:u8)
  n281 = Flatten To String(anything=w89, byte order (0:big-endian, network order)=2) -> (data string=w83:string)  [unwired: 2 in, 2 out]
  n282 = To Unsigned Byte Integer(number=w67) -> (unsigned 8bit integer=w70:u8)
  n283 = To Unsigned Byte Integer(number=w66) -> (unsigned 8bit integer=w69:u8)
  n284 = To Unsigned Byte Integer(number=w65) -> (unsigned 8bit integer=w68:u8)
  n285 = Flatten To String(anything=w88, byte order (0:big-endian, network order)=2) -> (data string=w84:string)  [unwired: 2 in, 2 out]
  n286 = Flatten To String(anything=w64, byte order (0:big-endian, network order)=2) -> (data string=w53:string)  [unwired: 2 in, 2 out]
  n287 = Flatten To String(anything=w68, byte order (0:big-endian, network order)=2) -> (data string=w59:string)  [unwired: 2 in, 2 out]
  n288 = Flatten To String(anything=w69, byte order (0:big-endian, network order)=2) -> (data string=w60:string)  [unwired: 2 in, 2 out]
  n289 = Flatten To String(anything=w70, byte order (0:big-endian, network order)=2) -> (data string=w62:string)  [unwired: 2 in, 2 out]
  n290 = Concatenate Strings(w51, w50, w49, w48, w47, w46, w45, w44) -> (w52:string)
  n291 = Concatenate Strings(w83, w84, w52) -> (w91:string)
  n292 = call "CRC_8_CCIT.vi"("Data String"=w91) -> ("Numeric"=w90:u8)  [unwired: 10 in]
  n293 = To Unsigned Byte Integer(number=w90) -> (unsigned 8bit integer=w93:u8)
  n294 = Exclusive Or(1:u8 85, 2:w93) -> (0:w92:u8)
  n295 = Flatten To String(anything=w92, byte order (0:big-endian, network order)=2) -> (data string=w61:string)  [unwired: 2 in, 2 out]
  n296 = String Length(string=w91) -> (length=w86:i32)
  n297 = To Unsigned Byte Integer(number=w86) -> (unsigned 8bit integer=w96:u8)
  n298 = Exclusive Or(1:w96, 2:u8 85) -> (0:w95:u8)
  n299 = Flatten To String(anything=w95, byte order (0:big-endian, network order)=2) -> (data string=w87:string)  [unwired: 2 in, 2 out]
  n300 = Concatenate Strings(w59, w60, w61, w62, w87, w83, w84, w52, w53) -> (w11:string)
  n301 = case shown="True" "StimInitializationEnable" {
    tunnel: "VISA resource name" -> [w576 w587]
    tunnel: w11 -> [_ w583]
    tunnel: ["" "Stimulation Started"] -> _
    tunnel: "error in (no error)" -> [w577 w581]
    tunnel: [w576 w580] -> w8
    tunnel: [w577 w579] -> w7
    frame False {
    }
    frame True {
      n302 = VISA Write(VISA resource name=w587, write buffer=w583, error in (no error)=w581) -> (VISA resource name out=w580:refnum<visa-resource-name>, return count=w585:u32, error out=w579:errorcluster)
      n303 = Equal?(x=w585, y=u32 0) -> (x = y?=→"Stimulation Started":bool)
    }
  }
  "VISA resource name out" <- w8
  "error out" <- w7
